vi "Trigger Detector (Unbalance).vi"(0 "unbalance":T4, 1 "reset? (F)":bool, 5 "triggers definition":T3(array[cluster]), 9 "data timestamp":timestamp, 11 "error in (no error)":errorcluster) -> (4 "triggers":T2(array[cluster]), 6 "actual trigger state":T1[](array[typedef]), 15 "error out":errorcluster)   [LabVIEW 2014, in "NI_EP_Power Quality.lvlib"]
doc: "Detects crossing of limits for the measurement that you specify and returns triggers if occur.\n\nThis VI supports measuring single-line and multiple-line systems except the DBL instance. Use the DBL instance to measure one channel on one line at one time."
uses:
  <vilib>/addons/Electrical Power/PQ/NI_EP_Power Quality.lvlib
  <vilib>/addons/Electrical Power/PQ/Common/Controls/ep_Trigger State.ctl
  <vilib>/addons/Electrical Power/PQ/Triggers/subVIs/ep_Trigger Definition.ctl
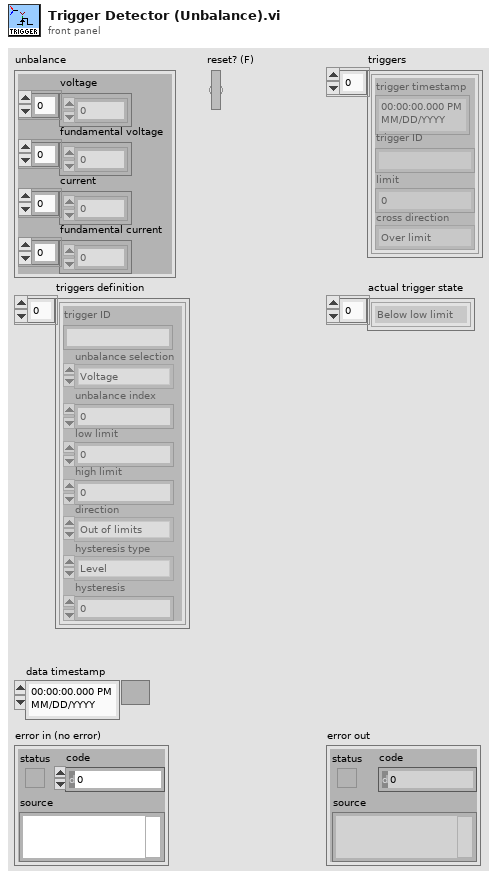
[diagram p1: front panel]
types:
  T1 = typedef "NI_EP_Power Quality.lvlib/ep_Trigger State.ctl" = enum16{"Below low limit", "In the limits", "Over high limit"}
  T2 = cluster{"trigger timestamp":timestamp, "trigger ID":string, "limit":dbl, "cross direction":enum16{"Over limit", "Below limit"}}[]
  T3 = cluster{"trigger ID":string, "unbalance selection":enum16{"Voltage", "Fundamental voltage", "Current", "Fundamental Current"}, "unbalance index":u32, "low limit":dbl, "high limit":dbl, "direction":enum16{"Out of limits", "Back to limits", "Both"}, "hysteresis type":enum16{"Level", "Time"}, "hysteresis":dbl}[]
  T4 = cluster{"voltage":dbl[], "fundamental voltage":dbl[], "current":dbl[], "fundamental current":dbl[]}
  T5 = cluster{"trigger time":timestamp, "trigger unique id":string, "limit":dbl, "cross direction":enum16{"Over limit", "Below limit"}}[]
  T6 = typedef "NI_EP_Power Quality.lvlib/ep_Trigger Definition.ctl" = cluster{"trigger ID":string, "low limit":dbl, "high limit":dbl, "direction":enum16{"Out of limits", "Back to limits", "Both"}, "hysteresis type":enum16{"Level", "Time"}, "hysteresis":dbl}
  T7 = cluster{"Lo in progr.":bool, "Hi in progr.":bool, "Lo trig. time":timestamp, "Hi trig. time":timestamp}[]
  T8 = enum16{"Out of limits", "Back to limits", "Both"}
  T9 = cluster{"Lo in progr.":bool, "Lo in progr.":bool, "data timestamp":timestamp, "data timestamp":timestamp}
  T10 = enum16{"Voltage", "Fundamental voltage", "Current", "Fundamental Current"}
  T11 = cluster{"Lo in progr.":bool, "Hi in progr.":bool, "Lo trig. time":timestamp, "Hi trig. time":timestamp}
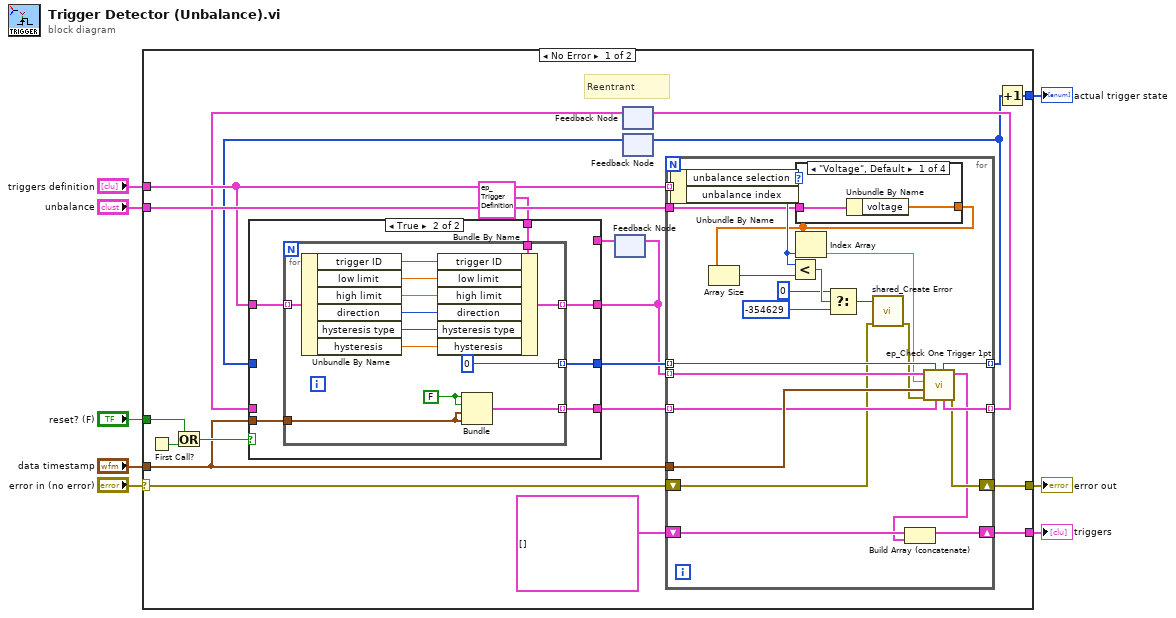
[diagram p0: block diagram]
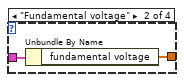
[diagram p3: hidden frame]
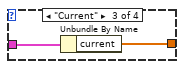
[diagram p4: hidden frame]
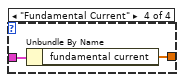
[diagram p5: hidden frame]
diagram:
  n1 = case shown="No Error" "error in (no error)" {
    selector: "error in (no error)" -> [w12 w82]
    tunnel: "unbalance" -> [w28 _]
    tunnel: "reset? (F)" -> [w26 _]
    tunnel: "triggers definition" -> [w24 _]
    tunnel: [w14 _] -> w7
    tunnel: "data timestamp" -> [w13 _]
    tunnel: [w11 w82] -> w8
    tunnel: [w9 _] -> w1
    frame No Error {
      # "Reentrant"
      n2 = First Call?() -> (First Call?: T/F=w27:bool)
      n3 = Or(x=w26, y=w27) -> (x .or. y?=w25:bool)
      n4 = feedback #1() -> (w17:T6[])  [unwired: 1 in]
      n5 = feedback #2() -> (w18:T7)  [unwired: 1 in]
      n6 = feedback #3() -> (w20:i8[])  [unwired: 1 in]
      n7 = case shown="True" w25 {
        tunnel: w24 -> [_ w37]
        tunnel: [w29 w36] -> w16
        tunnel: T6 {"trigger ID"="", "low limit"=0.0, "high limit"=0.0, "direction"=enum."Out of limits", "hysteresis type"=enum."Level", "hysteresis"=0.0} ("trigger definition") -> [_ w35]
        tunnel: [w31 w34] -> w22
        tunnel: [w30 w33] -> w21
        tunnel: w20 -> [w30 _]
        tunnel: w18 -> [w31 _]
        tunnel: w17 -> [w29 _]
        tunnel: w13 -> [_ w32]
        frame False {
        }
        frame True {
          n8 = for {
            tunnel: w37 -> [w46] mode=indexing
            tunnel: [w45] -> w36 mode=indexing
            tunnel: w35 -> [w44]
            tunnel: [w40] -> w34 mode=indexing
            tunnel: [i8 0] -> w33 mode=indexing
            tunnel: w32 -> [w41]
            w42 = FALSE ("Lo in progr.")
            n9 = Unbundle By Name(w46) -> ("trigger ID"=w49:string, "low limit"=w39:dbl, "high limit"=w38:dbl, "direction"=w48:T8, "hysteresis type"=w47:enum16{"Level", "Time"}, "hysteresis"=w50:dbl)
            n10 = Bundle By Name(cluster=w44, "trigger ID"=w49, "low limit"=w39, "high limit"=w38, "direction"=w48, "hysteresis type"=w47, "hysteresis"=w50) -> (w45:T6)
            n11 = Bundle("Lo in progr."=w42, "Lo in progr."=w42, "data timestamp"=w41, "data timestamp"=w41) -> (w40:T9)  [unwired: 1 in]
          }
        }
      }
      n12 = feedback-in #1(w16) -> ()
      n13 = for {
        tunnel: w13 -> [w68]
        tunnel: w24 -> [w66] mode=indexing
        tunnel: w28 -> [w57]
        tunnel: w22 -> [w65] mode=indexing
        tunnel: w21 -> [w70] mode=indexing
        tunnel: [w69] -> w10 mode=indexing
        tunnel: [w67] -> w19 mode=indexing
        tunnel: w16 -> [w73] mode=indexing
        shift-right: [w72] -> w14
        shift-left: T5 [] -> [w71]
        shift-right: [w64] -> w11
        shift-left: w12 -> [w52]
        n14 = Unbundle By Name(w66) -> ("unbalance selection"=w58:T10, "unbalance index"=w63:u32)
        n15 = case shown="\"Voltage\", Default" w58 {
          tunnel: w57 -> [w75 w77 w79 w81]
          tunnel: [w74 w76 w78 w80] -> w56
          frame "Voltage", Default {
            n16 = Unbundle By Name(w75) -> ("voltage"=w74:dbl[])
          }
          frame "Fundamental voltage" {
            n17 = Unbundle By Name(w77) -> ("fundamental voltage"=w76:dbl[])
          }
          frame "Current" {
            n18 = Unbundle By Name(w79) -> ("current"=w78:dbl[])
          }
          frame "Fundamental Current" {
            n19 = Unbundle By Name(w81) -> ("fundamental current"=w80:dbl[])
          }
        }
        n20 = Array Size(array=w56) -> (size(s)=w62:i32)
        n21 = Less?(x=w63, y=w62) -> (x < y?=w61:bool)
        n22 = Index Array(array=w56, index=w63) -> (element=w59:dbl)
        n23 = Select(t=0 ("error code (0)"), s=w61, f=-354629 ("error code (0)")) -> (s? t:f=w53:i32)
        n24 = call <vilib>:"shared_Create Error.vi"("error in (no error)"=w52, "error code (0)"=w53) -> ("error out"=w51:errorcluster)  [unwired: 9 in]
        n25 = call <vilib>:"ep_Check One Trigger 1pt.vi"("trig. local in"=w65, "prev. state in"=w70, "error in (no error)"=w51, "data time stamp"=w68, "value in"=w59, "trigger definition"=w73) -> ("error out"=w64:errorcluster, "triggers list"=w60:T5, "trig. local out"=w67:T11, "state out"=w69:i8)  [unwired: 2 in]
        n26 = Build Array (concatenate)(w71, w60) -> (w72:T5)
      }
      n27 = feedback-in #2(w19) -> ()
      n28 = feedback-in #3(w10) -> ()
      n29 = Increment(x=w10) -> (x+1=w9:i8[])
    }
    frame Error {
    }
  }
  "error out" <- w8
  "triggers" <- w7
  "actual trigger state" <- w1
